vi "Filter.vi"(0 "Array":dbl[](array[numeric]), 1 "init/cont (init:F)":bool) -> (2 "Decimated Array":dbl[](array[numeric]))   [LabVIEW 2017]
uses:
  <vilib>/Analysis/3filter.llb/Filter Passband Type.ctl
  <vilib>/Analysis/3filter.llb/Butterworth Filter (DBL).vi
  <vilib>/Analysis/2dsp.llb/Decimate (continuous, DBL).vi
  <vilib>/Analysis/NI_AALBase.lvlib
  <vilib>/Analysis/NI_AALPro.lvlib
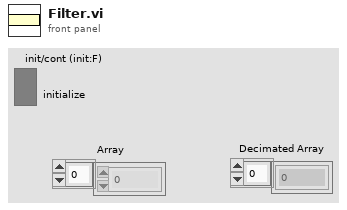
[diagram p1: front panel]
types:
  T1 = typedef "NI_AALBase.lvlib/Filter Passband Type.ctl" = enum32{"Lowpass", "Highpass", "Bandpass", "Bandstop"}
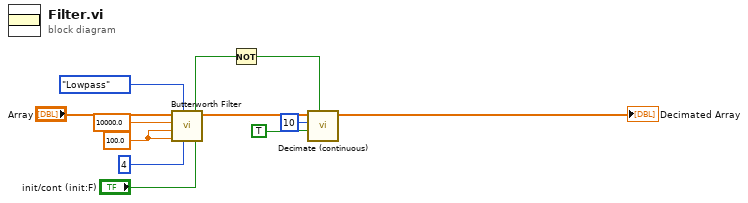
[diagram p0: block diagram]
diagram:
  w9 = 100.0 ("low cutoff freq: fl")
  n1 = call-poly <vilib>:"Butterworth Filter.vi"("init/cont (init:F)"="init/cont (init:F)", "order"=4, "filter type"=Filter_Passband_Type."Lowpass", "low cutoff freq: fl"=w9, "high cutoff freq: fh"=w9, "sampling freq: fs"=10000.0, "X"="Array") -> ("Filtered X"=w6:dbl[])  [unwired: 1 in, 1 out]
  n2 = Not(x="init/cont (init:F)") -> (.not. x?=w1:bool)
  n3 = call-poly <vilib>:"Decimate (continuous).vi"("reset"=w1, "averaging"=TRUE, "decimating factor"=10, "X"=w6) -> ("Decimated Array"=→"Decimated Array":dbl[])  [unwired: 6 in, 1 out]
